vi "MP-Reset.vi"(8 "error in (no error)":errorcluster, 9 "Hard Reset?":bool caption="Hard Reset? (def: F - Soft Reset)", 10 "Sample Frequency":T5, 11 "TCP config":T6 {"Write timeout" format="%dms"; "Read timeout" format="%dms"; "OC timeout" format="%dms"}) -> (0 "error out":errorcluster, 2 "System Status":T1={"System Type"=enum."MicroPulse 5", "Serial No."=0, "Channels"={"Conv"=0, "PA"=0, "Extra"=0}, "Sample Frequency"={"Default"=0, "Actual"=0}, "Software Versions"="", "Data Output Format"={"Default"=enum."8-bit Mode", "Actual"=enum."8-bit Mode"}, "Temperatures"={"System"=0, "Processor"=0, "Slave Sys"=0, "Slave Proc"=0}, "Tx Buffer Size"=0, "System Error"="", "No. of Cards"=0, "DAC Gain"=0, "Uptimes"={"since Power"=0, "since RSTS"=0, "since SRST"=0}, "Voltages"=[], "Interface Cards"=[]} {"Interface Cards"."FPGA - T" format="%.0f °C"; "Interface Cards"."Board - T" format="%.0f °C"; "Voltages"."Difference" format="%.2fV"; "Voltages"."Measured" format="%.2fV"; "Voltages"."Nominal" format="%.2fV"; "DAC Gain" format="%.0fdB"; "Tx Buffer Size" format="%.0fMB"; "Temperatures"."Slave Proc" format="%.0f C"; "Temperatures"."Slave Sys" format="%.0f C"; "Temperatures"."Processor" format="%.0f C"; "Temperatures"."System" format="%.0f C"; "Sample Frequency"."Actual" format="%.0fMHz"; "Sample Frequency"."Default" format="%.0fMHz"}, 3 "TCP config out":T6 {"Write timeout" format="%dms"; "Read timeout" format="%dms"; "OC timeout" format="%dms"})   [LabVIEW 2026, in "MicroPulse_Driver.lvlib"]
doc: "Performs either a hard or a soft reset of the Micropulse depending on the value of <b>Hard Reset?</b>\nOptionally allows for changing the sampling rate from the instrument's default.\nReturns the new settings data in <b>Micropulse Registry Out</b>."
uses:
  MicroPulse_Driver.lvlib
  Public/Data/Datatypes/TCP config.ctl
  Public/Data/Datatypes/MP - sample frequency.ctl
  Public/Data/Datatypes/MP - general system status.ctl
  <instrlib>/MicroPulse/Public/Data/Datatypes/MP - instrument type.ctl
  Public/Data/Datatypes/MP - data output format.ctl
  Public/Data/Datatypes/MP - interface card status.ctl
panel:
  out "Items left in buffer":string[](array[string])
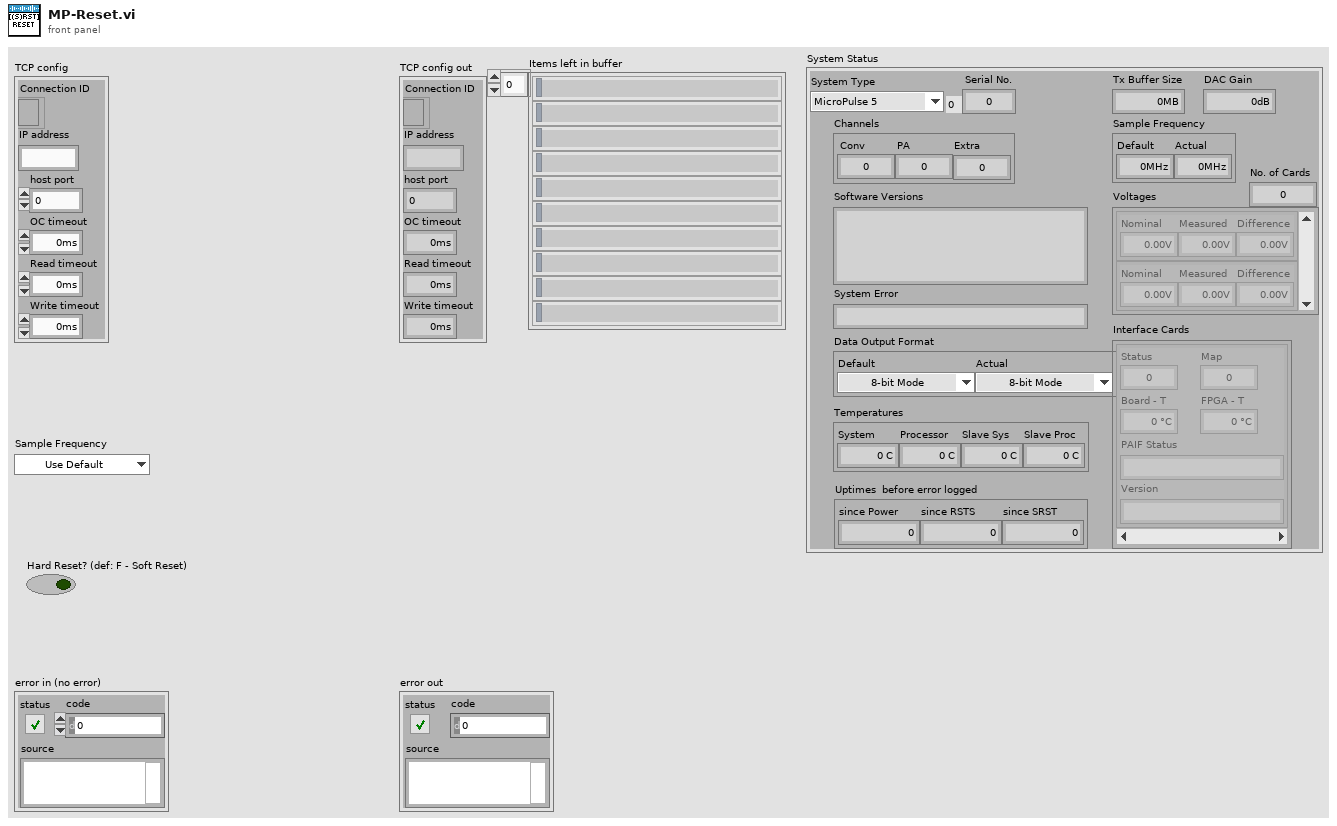
[diagram p1: front panel]
types:
  T1 = typedef "MicroPulse_Driver.lvlib/MP - general system status.ctl" = cluster{"System Type":T2, "Serial No.":u64, "Channels":cluster{"Conv":u8, "PA":u16, "Extra":u32}, "Sample Frequency":cluster{"Default":u8, "Actual":u8}, "Software Versions":string, "Data Output Format":cluster{"Default":T3, "Actual":T3}, "Temperatures":cluster{"System":u8, "Processor":u8, "Slave Sys":u8, "Slave Proc":u8}, "Tx Buffer Size":u32, "System Error":string, "No. of Cards":u8, "DAC Gain":i16, "Uptimes":cluster{"since Power":u32, "since RSTS":u32, "since SRST":u32}, "Voltages":cluster{"Nominal":dbl, "Measured":dbl, "Difference":dbl}[], "Interface Cards":T4[]}
  T2 = typedef "MicroPulse_Driver.lvlib/MP - instrument type.ctl" = enum16{"MicroPulse 5", "LT1", "LT2", "LTPA", "MPLT", "MicroPulse 6", "PipeScanner", "<MicroPulse>", "Micropulse 4", "Simulated Data"}
  T3 = typedef "MicroPulse_Driver.lvlib/MP - data output format.ctl" = enum16{"", "8-bit Mode", "10-bit Mode", "12-bit Mode", "16-bit Mode", "8-bit Log Mode", "12-bit Packed Mode"}
  T4 = typedef "MicroPulse_Driver.lvlib/MP - interface card status.ctl" = cluster{"Status":u8, "Map":u8, "Board - T":u8, "FPGA - T":u8, "PAIF Status":string, "Version":string}
  T5 = typedef "MicroPulse_Driver.lvlib/MP - sample frequency.ctl" = enum16{"Use Default", "200MHz (LT2 only)", "100MHz", "50MHz", "25MHz", "10MHz"}
  T6 = typedef "MicroPulse_Driver.lvlib/TCP config.ctl" = cluster{"Connection ID":refnum<k5>, "IP address":string, "host port":u16, "OC timeout":i32, "Read timeout":i32, "Write timeout":i32}
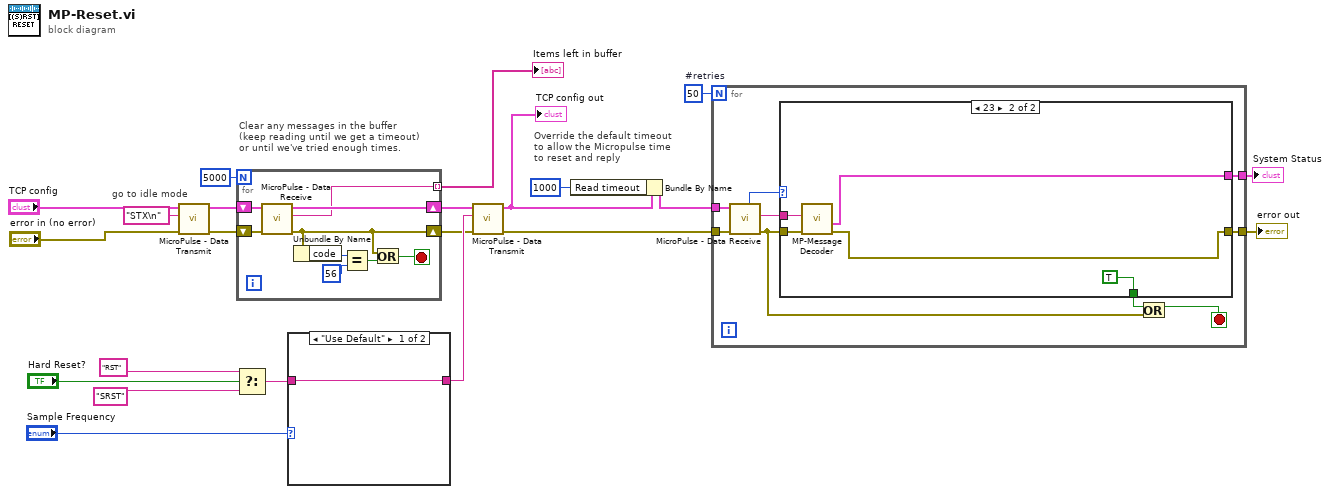
[diagram p0: block diagram]
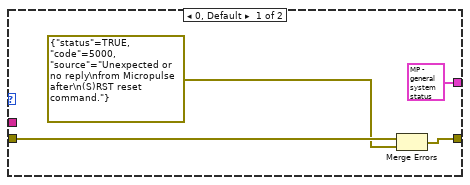
[diagram p2: hidden frame]
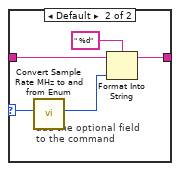
[diagram p3: hidden frame]
diagram:
  w2 = 50  # #retries
  # "go to idle mode"
  # "Clear any messages in the buffer\n(keep reading until we get a timeout)\nor until we've tried enough times."
  # "Override the default timeout\nto allow the Micropulse time\nto reset and reply"
  n1 = call "MicroPulse - Data Transmit.vi"("error in (no error)"="error in (no error)", "data"="STX\n", "TCP config"="TCP config") -> ("error out"=w9:errorcluster, "TCP config out"=w6:T6)  [unwired: 6 in, 1 out]
  n2 = for {
    N: 5000 -> [_]
    shift-right: [w30] -> w11
    shift-left: w6 -> [w31]
    shift-right: [w24] -> w10
    shift-left: w9 -> [w29]
    tunnel: [w25] -> w3 mode=indexing
    stop <- w23 stop-if-true
    n3 = call "MicroPulse - Data Receive.vi"("error in (no error)"=w29, "TCP config"=w31) -> ("error out"=w24:errorcluster, "data message"=w25:string, "TCP config out"=w30:T6)  [unwired: 4 in, 3 out]
    n4 = Unbundle By Name(w24) -> ("code"=w28:i32)
    n5 = Equal?(x=w28, y=56) -> (x = y?=w26:bool)
    n6 = Or(x=w24, y=w26) -> (x .or. y?=w23:bool)
  }
  "Items left in buffer" <- w3
  n7 = Select(t="RST" ("data"), s="Hard Reset?", f="SRST" ("data")) -> (s? t:f=w14:string)
  n8 = case shown="\"Use Default\"" "Sample Frequency" {
    selector: "Sample Frequency" -> [_ w36]
    tunnel: w14 -> [w32 w37]
    tunnel: [w32 w35] -> w13
    frame "Use Default" {
    }
    frame Default {
      # "add the optional field\nto the command"
      n9 = call "Convert Sample Rate MHz to and from Enum.vi"("Sample Frequency enum in"=w36) -> ("MHz out"=w33:u8)  [unwired: 9 in, 1 out]
      n10 = Format Into String(format string=" %d", initial string=w37, w33) -> (resulting string=w35:string)  [unwired: 1 in, 1 out]
    }
  }
  n11 = call "MicroPulse - Data Transmit.vi"("error in (no error)"=w10, "data"=w13, "TCP config"=w11) -> ("error out"=w22:errorcluster, "TCP config out"=w15:T6)  [unwired: 6 in, 1 out]
  "TCP config out" <- w15
  n12 = Bundle By Name(cluster=w15, "Read timeout"=1000) -> (w21:T6)
  n13 = for {
    N: w2 -> [_]
    tunnel: w21 -> [w45]
    tunnel: w22 -> [w46]
    tunnel: [w41] -> w19
    tunnel: [w42] -> w1
    stop <- w39 stop-if-true
    n14 = call "MicroPulse - Data Receive.vi"("error in (no error)"=w46, "TCP config"=w45) -> ("error out"=w38:errorcluster, "data message"=w44:string, "Header Byte"=w43:u8)  [unwired: 4 in, 3 out]
    n15 = case shown="23" w43 {
      tunnel: w44 -> [_ w55]
      tunnel: w38 -> [w50 w54]
      tunnel: [T1 {"System Type"=enum."MicroPulse 5", "Serial No."=0, "Channels"={"Conv"=0, "PA"=0, "Extra"=0}, "Sample Frequency"={"Default"=0, "Actual"=0}, "Software Versions"="", "Data Output Format"={"Default"=enum."8-bit Mode", "Actual"=enum."8-bit Mode"}, "Temperatures"={"System"=0, "Processor"=0, "Slave Sys"=0, "Slave Proc"=0}, "Tx Buffer Size"=0, "System Error"="", "No. of Cards"=0, "DAC Gain"=0, "Uptimes"={"since Power"=0, "since RSTS"=0, "since SRST"=0}, "Voltages"=[], "Interface Cards"=[]} ("System Status") w51] -> w42
      tunnel: [w49 w53] -> w41
      tunnel: [_ TRUE] -> w40
      frame 0, Default {
        n16 = Merge Errors(w50, errorcluster {"status"=TRUE, "code"=5000, "source"="Unexpected or no reply\nfrom Micropulse after\n(S)RST reset command."} ("error in")) -> (w49:errorcluster)
      }
      frame 35 {
        n17 = call "MP-Message Decoder.vi"("error in (no error)"=w54, "SDO messages"=w55) -> ("error out"=w53:errorcluster, "System Status"=w51:T1)  [unwired: 3 in, 5 out]
      }
    }
    n18 = Or(x=w40, y=w38) -> (x .or. y?=w39:bool)
  }
  "error out" <- w19
  "System Status" <- w1
